vi "Send_zero_DC.vi"(8 "error in (no error)":errorcluster, 11 "machine":T1 {"TimeStamp" format="%.2f"}) -> (0 "error out":errorcluster, 3 "String":string)   [LabVIEW 2020]
uses:
  DataSocketCluster external.ctl
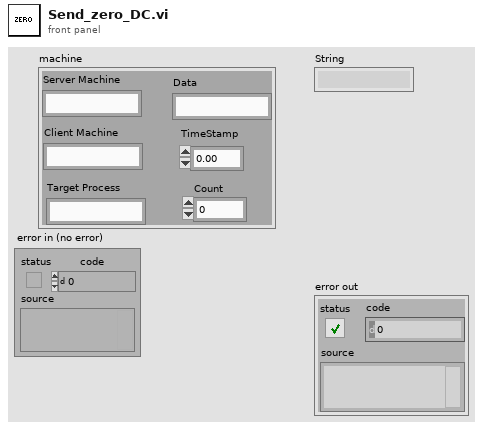
[diagram p1: front panel]
types:
  T1 = typedef "DataSocketCluster external.ctl" = cluster{"Server Machine":string, "Client Machine":string, "Data":string, "TimeStamp":dbl, "Count":i32, "Target Process":string}
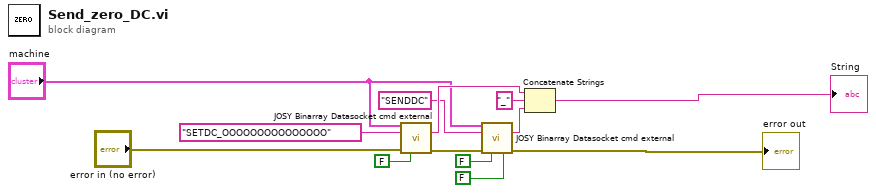
[diagram p0: block diagram]
diagram:
  n1 = call "JOSY Binarray Datasocket cmd external.vi"("DataSocketCluster In"="machine", "Command"="SETDC_OOOOOOOOOOOOOOO" ("DC-String 2"), "error in (no error)"="error in (no error)", "Command has variable"=FALSE) -> ("Reply data"=w12:string, "error out"=w4:errorcluster)  [unwired: 8 in, 2 out]
  n2 = call "JOSY Binarray Datasocket cmd external.vi"("DataSocketCluster In"="machine", "Command"="SENDDC", "error in (no error)"=w4, "Command has variable"=FALSE, "String"=FALSE) -> ("Reply data"=w11:string, "error out"=→"error out":errorcluster)  [unwired: 7 in, 2 out]
  n3 = Concatenate Strings(w12, "_" ("string"), w11) -> (→"String":string)
